vi "ToString.vi"(8 "error in (no error)":errorcluster, 11 "Ring D Element in":refnum<class "String dropdown D Element.lvclass">) -> (0 "error out":errorcluster, 2 "String":string, 3 "Ring D Element out":refnum<class "String dropdown D Element.lvclass">)   [LabVIEW 2018, in "D Datagrid Library.lvlib" / "String dropdown D Element.lvclass"]
uses:
  String dropdown D Element.lvclass
  String dropdown D Element.lvclass/String dropdown D Element.ctl
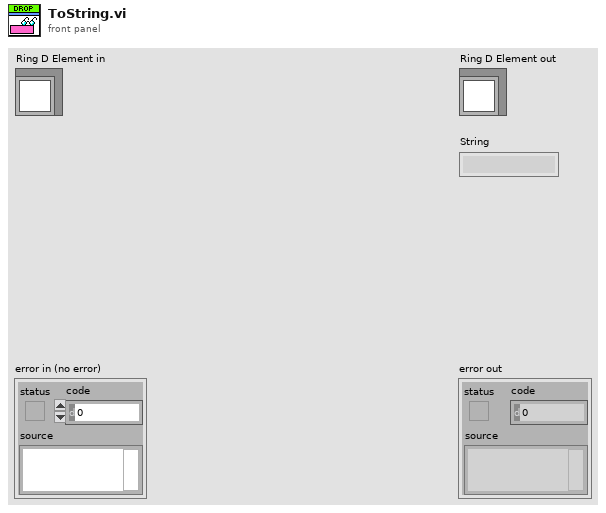
[diagram p1: front panel]
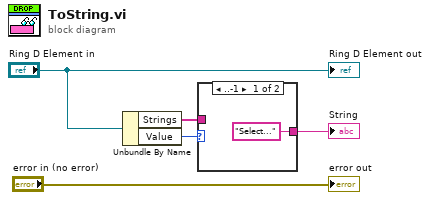
[diagram p0: block diagram]
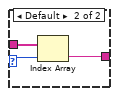
[diagram p2: hidden frame]
diagram:
  n1 = Unbundle By Name("Ring D Element in") -> ("Strings"=w3:string[], "Value"=w2:i32)
  n2 = case shown="..-1" w2 {
    selector: w2 -> [_ w8]
    tunnel: w3 -> [_ w9]
    tunnel: ["Select..." ("String") w7] -> w1
    frame ..-1 {
    }
    frame Default {
      n3 = Index Array(array=w9, index=w8) -> (element=w7:string)
    }
  }
  "String" <- w1
  "error out" <- "error in (no error)"
  "Ring D Element out" <- "Ring D Element in"
